vi "FollowPath.vi"(1 "Parameter String":string, 2 "Reinit":bool) -> (0 "Increment":bool)   [LabVIEW 2018]
uses:
  sensors.vi
  refnums.vi
  <vilib>/Rock Robotics/WPI/Utilities/WPI_GetSetVariantRefNum.vi
  dsinstructions.vi
panel:
  out "FF Contribution":dbl
  out "Speed PID Tracking":cluster{"Goal Wheel Position":dbl, dbl}(graph)={"Goal Wheel Position"=0.0, -90.17571233858979}
  out "Speed Contribution Tracking":cluster{dbl, dbl, dbl}(graph)
  in  "N-Int Speed":i32=5 caption="N-Int"
  in  "N-Diff Speed":i32=10 caption="N-Diff"
  in  "Kd Speed":dbl=0.005
  in  "Ki Speed":dbl=0.1
  in  "Kp Speed":dbl=0.01
  out "Robot Position":cluster{dbl[], dbl[]}[](graph)
  in  "Plot":bool
  in  "N-Int Turning":i32=10 caption="N-Int"
  in  "N-Diff Turning":i32=10 caption="N-Diff"
  in  "Kd Turning":dbl=0.01
  in  "Ki Turning":dbl=0.1
  in  "Kp Turning":dbl=0.05
  out "Turning PID Tracking":cluster{"Goal Wheel Position":dbl, dbl}(graph)={"Goal Wheel Position"=0.0, -90.17571233858979}
  out "Turning Contribution Tracking":cluster{dbl, dbl, dbl}(graph)
  in  "Manual Control":bool
  in  "Look-Ahead Time (s)":dbl=0.25
  in  "Search Window (s)":dbl=2.0
  # "Orientation Control"
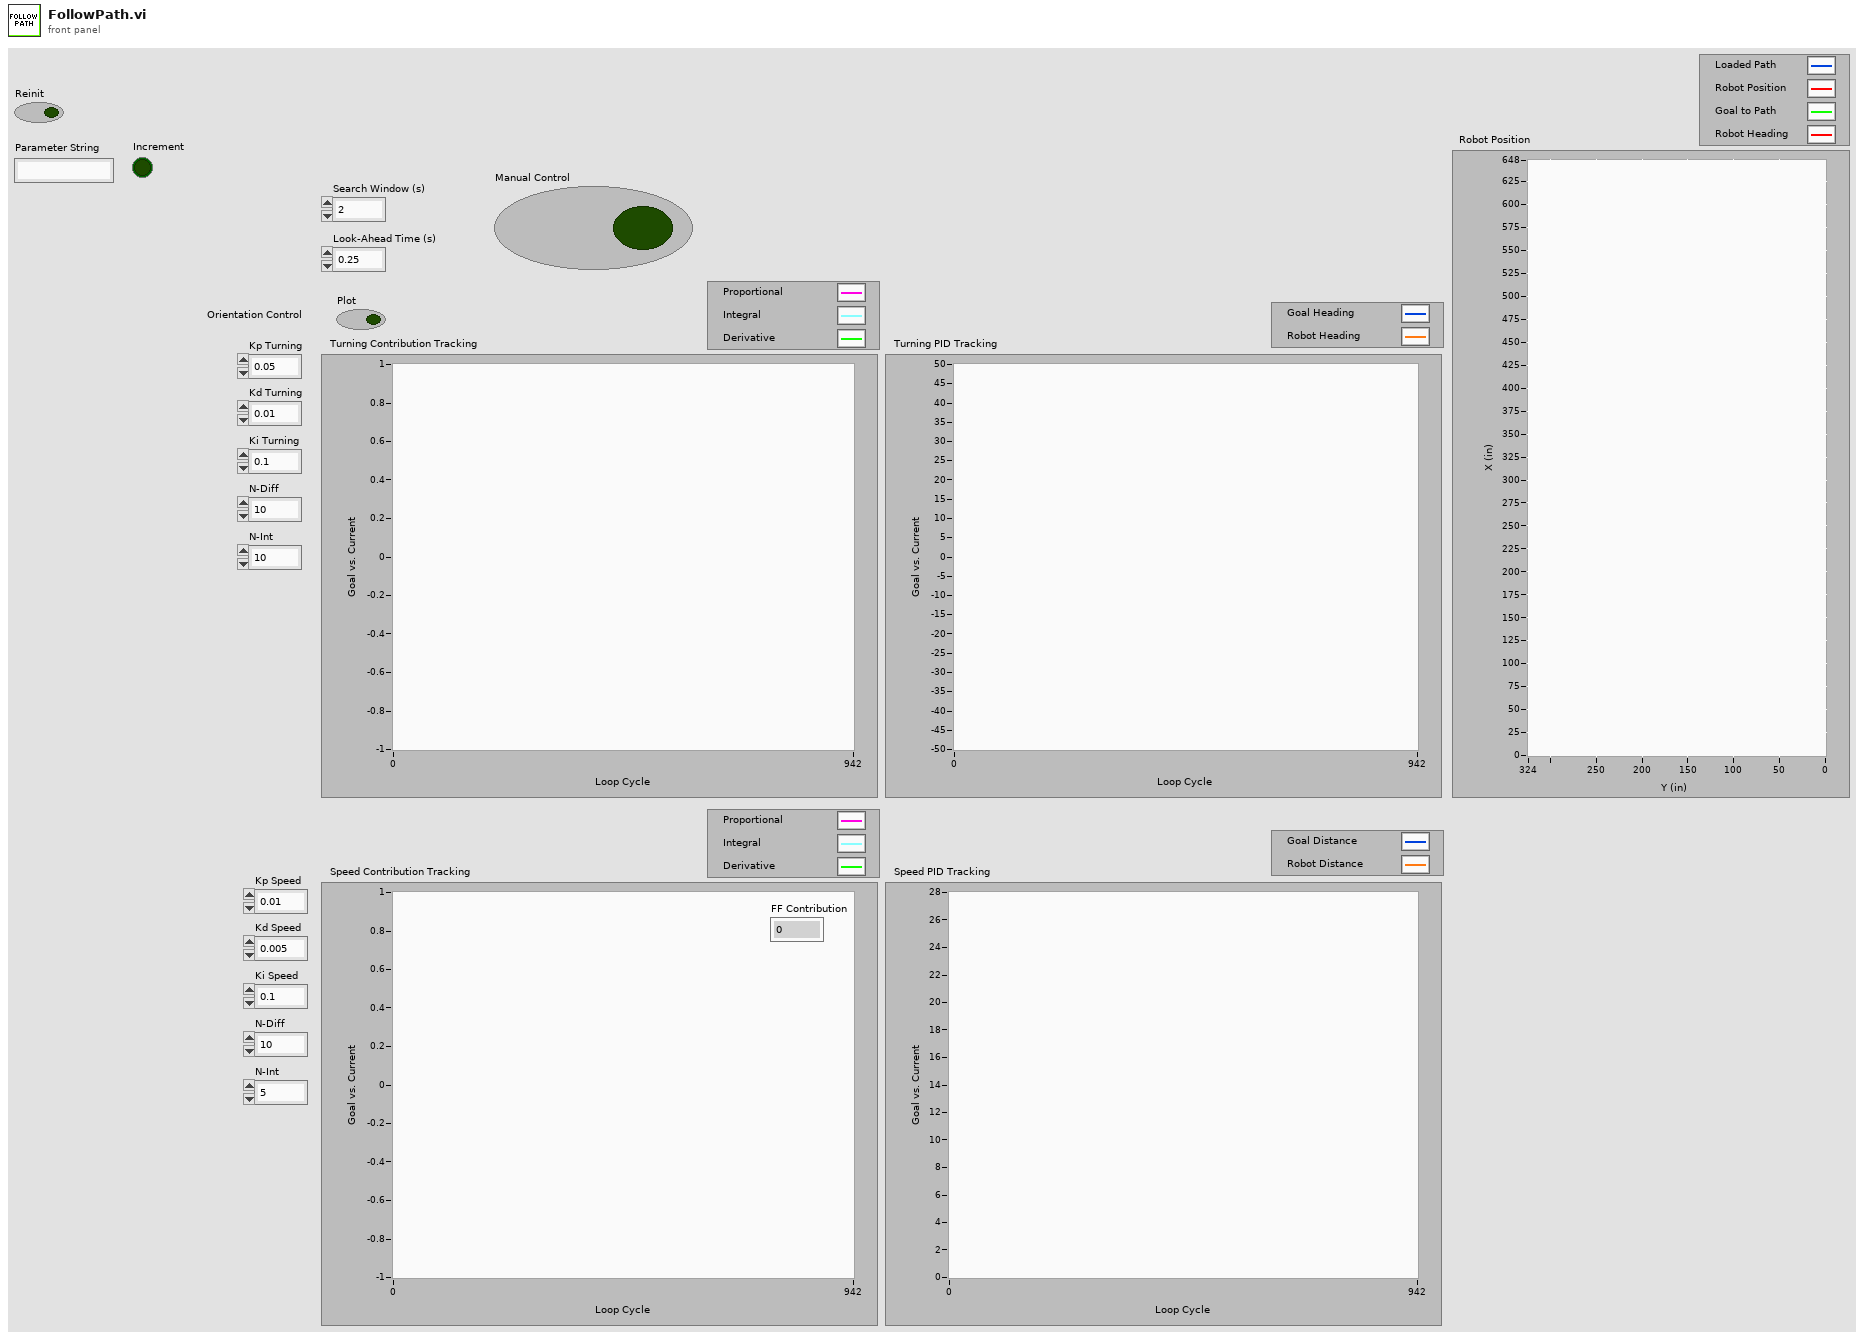
[diagram p1: front panel]
types:
  T1 = typedef "WPI_JoystickDevRef.ctl" = cluster{"Device":T2}
  T2 = typedef "WPI_JoystickDeviceEnum.ctl" = enum16{"USB 0", "USB 1", "USB 2", "USB 3", "USB 4", "USB 5"}
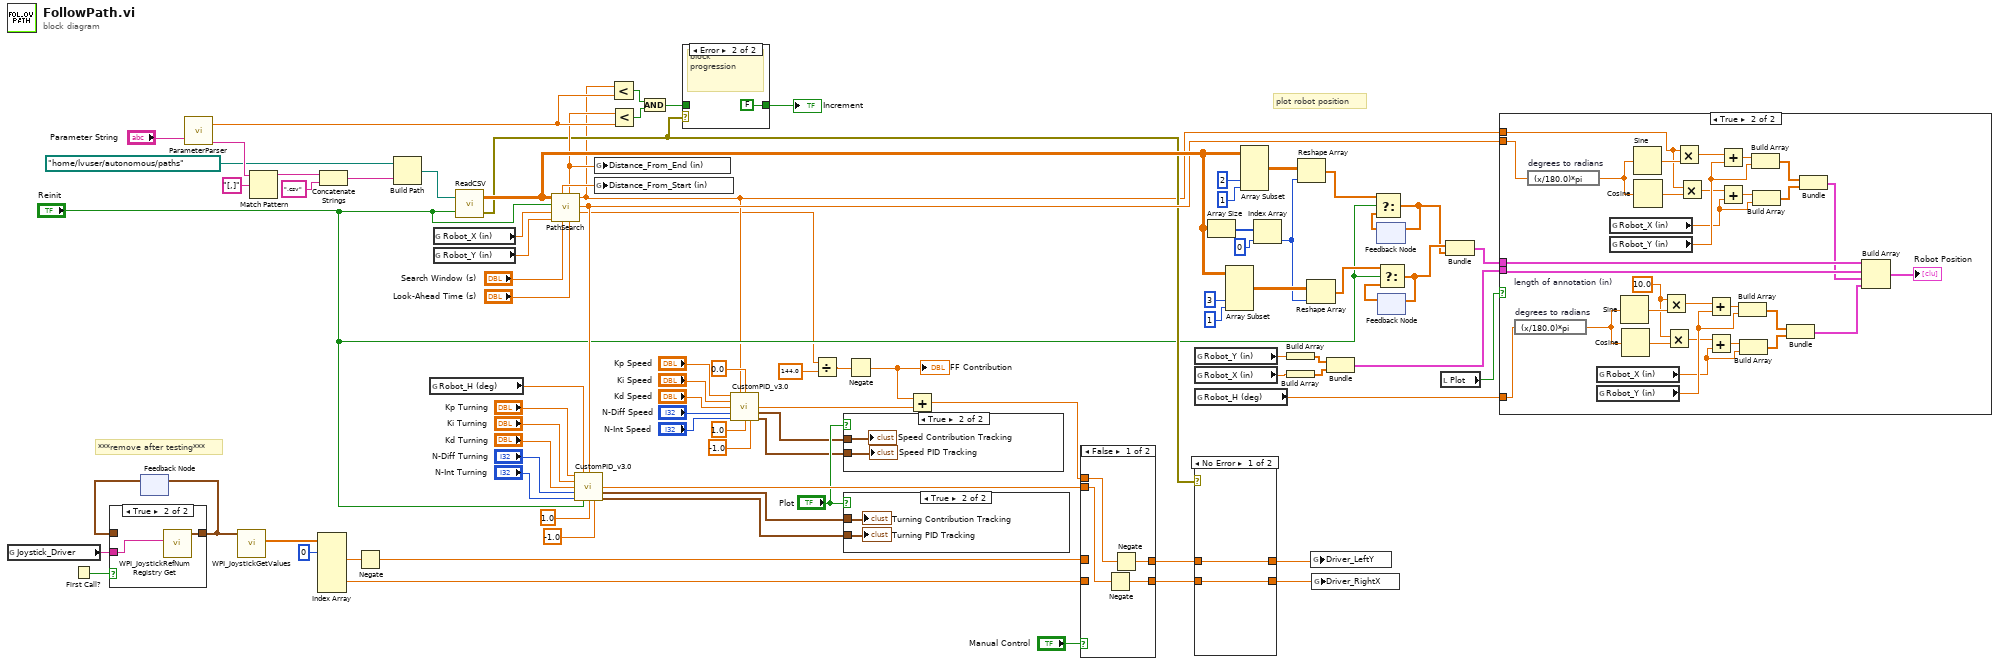
[diagram p0: block diagram]
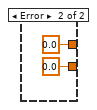
[diagram p4: hidden frame]
diagram:
  # "***remove after testing***"
  # "plot robot position"
  n1 = global read "refnums.vi" "Joystick_Driver"() -> (w76:string)
  n2 = First Call?() -> (First Call?: T/F=w79:bool)
  n3 = feedback #1() -> (w78:T1)  [unwired: 1 in]
  n4 = case shown="True" w79 {
    tunnel: [w90 w92] -> w77
    tunnel: w78 -> [w90 _]
    tunnel: w76 -> [_ w91]
    frame False {
    }
    frame True {
      n5 = call <vilib>:"WPI_JoystickRefNum Registry Get.vi"("refnum name"=w91) -> ("JoystickDevRef"=w92:T1)  [unwired: 9 in, 1 out]
    }
  }
  n6 = feedback-in #1(w77) -> ()
  n7 = call "ParameterParser.vi"("Parameter String"="Parameter String") -> ("Remaining Parameter String"=w87:string, "Parameter"=w32:dbl)  [unwired: 1 in]
  n8 = call <vilib>:"WPI_JoystickGetValues.vi"("JoystickDevRef"=w77) -> ("Axes"=w75:dbl[])  [unwired: 6 in, 4 out]
  n9 = Match Pattern(string=w87, regular expression="[,]") -> (before substring=w22:string)  [unwired: 1 in, 3 out]
  n10 = Index Array(array=w75, index #1=0 ("index")) -> (element #2=w73:dbl, element #5=w71:dbl)  [unwired: 5 in, 4 out]
  n11 = Concatenate Strings(w22, ".csv" ("string")) -> (w21:string)
  n12 = Negate(x=w73) -> (-x=w72:dbl)
  n13 = Build Path(base path=path "/home/lvuser/autonomous/paths" ("path"), name or relative path=w21) -> (appended path=w85:path)
  n14 = global read "sensors.vi" "Robot_H (deg)"() -> (w69:dbl)
  n15 = global read "sensors.vi" "Robot_X (in)"() -> (w83:dbl)
  n16 = global read "sensors.vi" "Robot_Y (in)"() -> (w82:dbl)
  n17 = call "ReadCSV.vi"("Reinit"="Reinit", "File Path (.csv)"=w85) -> ("File Open Eror"=w26:errorcluster, "Data (index by row)"=w46:dbl[][])
  n18 = call "PathSearch.vi"("Look-Ahead Time (s)"="Look-Ahead Time (s)", "Search Window (s)"="Search Window (s)", "Robot Y (in)"=w82, "Robot X (in)"=w83, "Reint"="Reinit", "Path"=w46) -> ("Velocity Goal (in/s)"=w3:dbl, "Angle To Goal (deg)"=w33:dbl, "Distance to Goal (in)"=w17:dbl, "Distance from End (in)"=w31:dbl, "Distance from Start (in)"=w84:dbl)  [unwired: 1 out]
  n19 = call "CustomPID_v3.0.vi"("Kp"="Kp Turning", "Process Variable"=w69, "Goal"=w33, "Ki"="Ki Turning", "Kd"="Kd Turning", "N-Diff"="N-Diff Turning", "N-Int"="N-Int Turning", "Reinit"="Reinit", "Max Ouput"=1.0, "Min Output"=-1.0) -> ("Command"=w68:dbl, "Contribution Tracking"=w67:cluster{dbl, dbl, dbl}, "PID Tracking"=w66:cluster{"Goal Wheel Position":dbl, dbl})  [unwired: 2 in, 1 out]
  n20 = global write "sensors.vi" "Distance_From_End (in)"(w31) -> ()
  n21 = global write "sensors.vi" "Distance_From_Start (in)"(w84) -> ()
  n22 = Less?(x=w17, y=w32) -> (x < y?=w48:bool)
  n23 = Less?(x=w31, y=w32) -> (x < y?=w47:bool)
  n24 = And(x=w48, y=w47) -> (x .and. y?=w25:bool)
  n25 = case shown="Error" w26 {
    tunnel: [w93 FALSE] -> w24
    tunnel: w25 -> [w93 _]
    frame No Error {
    }
    frame Error {
      # "block progression"
    }
  }
  "Increment" <- w24
  n26 = call "CustomPID_v3.0.vi"("Kp"="Kp Speed", "Process Variable"=w17, "Goal"=0.0, "Ki"="Ki Speed", "Kd"="Kd Speed", "N-Diff"="N-Diff Speed", "N-Int"="N-Int Speed", "Max Ouput"=1.0, "Min Output"=-1.0) -> ("Command"=w6:dbl, "Contribution Tracking"=w8:cluster{dbl, dbl, dbl}, "PID Tracking"=w7:cluster{"Goal Wheel Position":dbl, dbl})  [unwired: 3 in, 1 out]
  n27 = Divide(x=w3, y=144.0) -> (x/y=w4:dbl)
  n28 = case shown="True" "Plot" {
    tunnel: w8 -> [_ w96]
    tunnel: w7 -> [_ w95]
    frame False {
    }
    frame True {
      "Speed Contribution Tracking" <- w96
      "Speed PID Tracking" <- w95
    }
  }
  n29 = case shown="True" "Plot" {
    tunnel: w67 -> [_ w98]
    tunnel: w66 -> [_ w97]
    frame False {
    }
    frame True {
      "Turning Contribution Tracking" <- w98
      "Turning PID Tracking" <- w97
    }
  }
  n30 = Negate(x=w4) -> (-x=w1:dbl)
  "FF Contribution" <- w1
  n31 = Add(x=w1, y=w6) -> (x+y=w5:dbl)
  n32 = case shown="False" "Manual Control" {
    tunnel: [w99 w104] -> w30
    tunnel: w72 -> [_ w104]
    tunnel: w71 -> [_ w103]
    tunnel: [w101 w103] -> w28
    tunnel: w68 -> [w102 _]
    tunnel: w5 -> [w100 _]
    frame False {
      n33 = Negate(x=w102) -> (-x=w101:dbl)
      n34 = Negate(x=w100) -> (-x=w99:dbl)
    }
    frame True {
    }
  }
  n35 = global read "sensors.vi" "Robot_Y (in)"() -> (w45:dbl)
  n36 = global read "sensors.vi" "Robot_X (in)"() -> (w44:dbl)
  n37 = global read "sensors.vi" "Robot_H (deg)"() -> (w23:dbl)
  n38 = case shown="No Error" w26 {
    tunnel: [w106 0.0] -> w29
    tunnel: w30 -> [w106 _]
    tunnel: [w105 0.0 ("upper limit")] -> w27
    tunnel: w28 -> [w105 _]
    frame No Error {
    }
    frame Error {
    }
  }
  n39 = Array Size(array=w46) -> (size(s)=w51:i32[])
  n40 = Array Subset(array=w46, index (col)=3 ("index"), length (col)=1 ("length")) -> (w52:dbl[][])  [unwired: 2 in]
  n41 = Array Subset(array=w46, index (col)=2 ("index"), length (col)=1 ("length")) -> (w54:dbl[][])  [unwired: 2 in]
  n42 = Index Array(array=w51, index=0) -> (element=w49:i32)
  n43 = Build Array(w45) -> (w42:dbl[])
  n44 = Build Array(w44) -> (w43:dbl[])
  n45 = Reshape Array(w54, w49) -> (w35:dbl[])
  n46 = Reshape Array(w52, w49) -> (w53:dbl[])
  n47 = global write "dsinstructions.vi" "Driver_LeftY"(w29) -> ()
  n48 = global write "dsinstructions.vi" "Driver_RightX"(w27) -> ()
  n49 = Bundle(w42, w43) -> (w37:cluster{dbl[], dbl[]})  [unwired: 1 in]
  n50 = feedback #2() -> (w39:dbl[])  [unwired: 1 in]
  n51 = Select(t=w35, s="Reinit", f=w39) -> (s? t:f=w40:dbl[])
  n52 = feedback-in #2(w40) -> ()
  n53 = feedback #3() -> (w38:dbl[])  [unwired: 1 in]
  n54 = Select(t=w53, s="Reinit", f=w38) -> (s? t:f=w41:dbl[])
  n55 = feedback-in #3(w41) -> ()
  n56 = local read "Plot"() -> (w34:bool)
  n57 = Bundle(w41, w40) -> (w36:cluster{dbl[], dbl[]})  [unwired: 1 in]
  n58 = case shown="True" w34 {
    tunnel: w37 -> [_ w138]
    tunnel: w36 -> [_ w137]
    tunnel: w17 -> [_ w125]
    tunnel: w33 -> [_ w124]
    tunnel: w23 -> [_ w111]
    frame False {
    }
    frame True {
      w110 = 10.0  # length of annotation (in)
      n59 = expression code="(x/180.0)*pi" "degrees to radians"(w111) -> (w112:dbl)
      n60 = expression code="(x/180.0)*pi" "degrees to radians"(w124) -> (w126:dbl)
      n61 = global read "sensors.vi" "Robot_X (in)"() -> (w121:dbl)
      n62 = global read "sensors.vi" "Robot_Y (in)"() -> (w122:dbl)
      n63 = global read "sensors.vi" "Robot_X (in)"() -> (w135:dbl)
      n64 = global read "sensors.vi" "Robot_Y (in)"() -> (w136:dbl)
      n65 = Sine(x=w112) -> (sin(x)=w113:dbl)
      n66 = Cosine(x=w112) -> (cos(x)=w114:dbl)
      n67 = Sine(x=w126) -> (sin(x)=w127:dbl)
      n68 = Cosine(x=w126) -> (cos(x)=w128:dbl)
      n69 = Multiply(x=w110, y=w113) -> (x*y=w115:dbl)
      n70 = Multiply(x=w110, y=w114) -> (x*y=w116:dbl)
      n71 = Multiply(x=w125, y=w127) -> (x*y=w129:dbl)
      n72 = Multiply(x=w125, y=w128) -> (x*y=w130:dbl)
      n73 = Add(x=w115, y=w122) -> (x+y=w117:dbl)
      n74 = Add(x=w116, y=w121) -> (x+y=w118:dbl)
      n75 = Add(x=w129, y=w136) -> (x+y=w131:dbl)
      n76 = Add(x=w130, y=w135) -> (x+y=w132:dbl)
      n77 = Build Array(w117, w122) -> (w119:dbl[])
      n78 = Build Array(w118, w121) -> (w120:dbl[])
      n79 = Build Array(w131, w136) -> (w133:dbl[])
      n80 = Build Array(w132, w135) -> (w134:dbl[])
      n81 = Bundle(w119, w120) -> (w109:cluster{dbl[], dbl[]})  [unwired: 1 in]
      n82 = Bundle(w133, w134) -> (w123:cluster{dbl[], dbl[]})  [unwired: 1 in]
      n83 = Build Array(w137, w138, w123, w109) -> (→"Robot Position":cluster{dbl[], dbl[]}[])
    }
  }
